vi "Util_App_CreateTempDirectory.vi"(1 "TempFolderPath":path) -> (0 "TempFolderPath_out":path)   [LabVIEW 2013]
panel:
  out "error out":errorcluster
  in  "error in":errorcluster
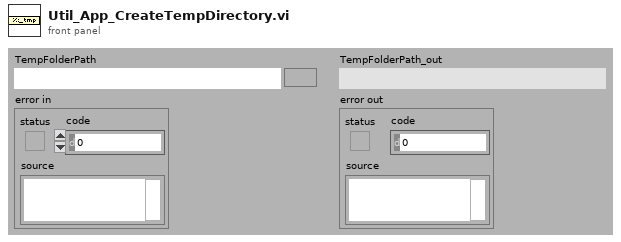
[diagram p1: front panel]
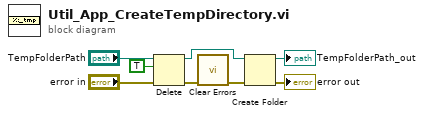
[diagram p0: block diagram]
diagram:
  n1 = Delete(path (use dialog)="TempFolderPath", entire hierarchy (F)=TRUE, error in="error in") -> (deleted path=w4:path, error out=w6:errorcluster)  [unwired: 2 in, 1 out]
  n2 = call <vilib>:"Clear Errors.vi"("error in (no error)"=w6) -> ("error out"=w5:errorcluster)  [unwired: 6 in]
  n3 = Create Folder(path (use dialog)=w4, error in=w5) -> (created path=→"TempFolderPath_out":path, error out=→"error out":errorcluster)  [unwired: 1 in, 1 out]
